vi "Convert Supported Color to .NET Color.vi"(8 "error in (no error)":errorcluster, 11 "Text Color":T1) -> (0 "error out":errorcluster, 3 ".NET Color":refnum<k24>)   [LabVIEW 2021, in "Rich Text Box.lvlib"]
uses:
  Rich Text Box.lvlib
  Text Colors.ctl
  System.Drawing
panel:
  # "see the License on the block diagram (Ctrl+E or Window:Show Block Diagram)"
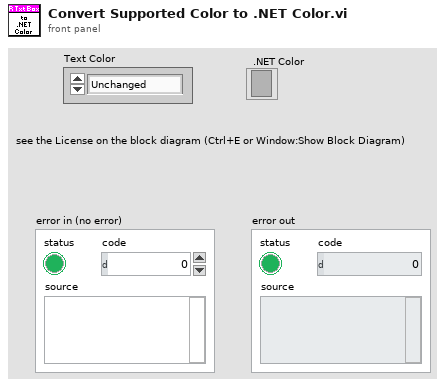
[diagram p1: front panel]
types:
  T1 = typedef "Rich Text Box.lvlib/Text Colors.ctl" = enum16{"Unchanged", "Black", "Blue", "Cyan", "Maroon", "Gray", "Violet", "Green", "Light Green", "Orange", "Yellow", "Magenta", "Red", "White"}
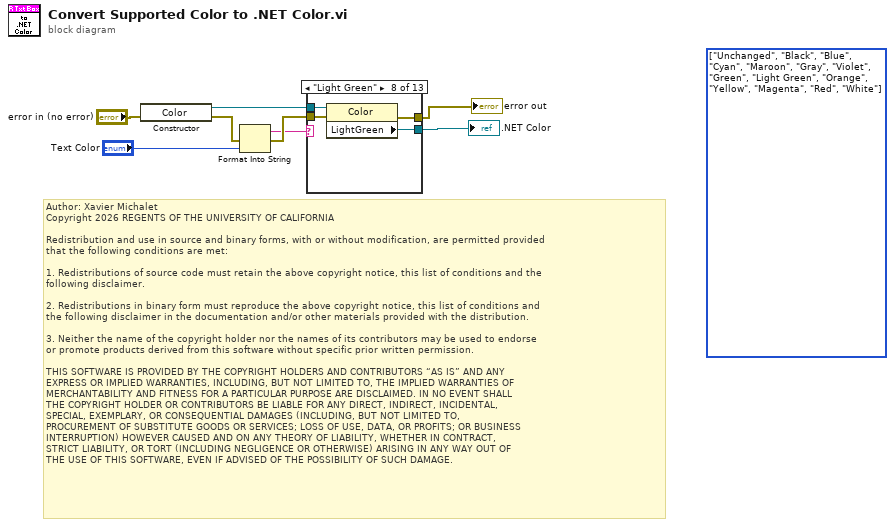
[diagram p0: block diagram]
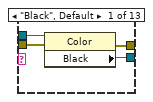
[diagram p2: hidden frame]
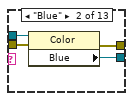
[diagram p3: hidden frame]
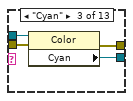
[diagram p4: hidden frame]
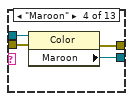
[diagram p5: hidden frame]
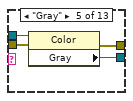
[diagram p6: hidden frame]
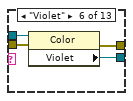
[diagram p7: hidden frame]
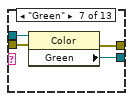
[diagram p8: hidden frame]
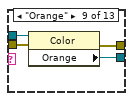
[diagram p9: hidden frame]
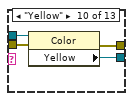
[diagram p10: hidden frame]
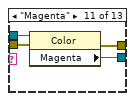
[diagram p11: hidden frame]
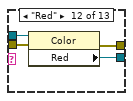
[diagram p12: hidden frame]
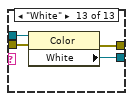
[diagram p13: hidden frame]
diagram:
  (unwired) T1[] [enum."Unchanged", enum."Black", enum."Blue", enum."Cyan", enum."Maroon", enum."Gray", enum."Violet", enum."Green", enum."Light Green", enum."Orange", enum."Yellow", enum."Magenta", enum."Red", enum."White"] items=["Unchanged", "Black", "Blue", "Cyan", "Maroon", "Gray", "Violet", "Green", "Light Green", "Orange", "Yellow", "Magenta", "Red", "White"] ("Array")
  # "Author: Xavier Michalet\nCopyright 2026 REGENTS OF THE UNIVERSITY OF CALIFORNIA\n\nRedistribution and use in source and binary forms, with or without modification, are permitted provided\nthat the following conditions are met:\n\n1. Redistributions of source code must retain the above copyright notice, this list of conditions and the\nfollowing disclaimer.\n\n2. Redistributions in binary form must reproduce the above copyright notice, this list of conditions and\nthe following disclaimer in the documentation and/or other materials provided with the distribution.\n\n3. Neither the name of the copyright holder nor the names of its contributors may be used to endorse \nor promote products derived from this software without specific prior written permission.\n\nTHIS SOFTWARE IS PROVIDED BY THE COPYRIGHT HOLDERS AND CONTRIBUTORS “AS IS” AND ANY \nEXPRESS OR IMPLIED WARRANTIES, INCLUDING, BUT NOT LIMITED TO, THE IMPLIED WARRANTIES OF\nMERCHANTABILITY AND FITNESS FOR A PARTICULAR PURPOSE ARE DISCLAIMED. IN NO EVENT SHALL\nTHE COPYRIGHT HOLDER OR CONTRIBUTORS BE LIABLE FOR ANY DIRECT, INDIRECT, INCIDENTAL, \nSPECIAL, EXEMPLARY, OR CONSEQUENTIAL DAMAGES (INCLUDING, BUT NOT LIMITED TO, \nPROCUREMENT OF SUBSTITUTE GOODS OR SERVICES; LOSS OF USE, DATA, OR PROFITS; OR BUSINESS\nINTERRUPTION) HOWEVER CAUSED AND ON ANY THEORY OF LIABILITY, WHETHER IN CONTRACT, \nSTRICT LIABILITY, OR TORT (INCLUDING NEGLIGENCE OR OTHERWISE) ARISING IN ANY WAY OUT OF\nTHE USE OF THIS SOFTWARE, EVEN IF ADVISED OF THE POSSIBILITY OF SUCH DAMAGE."
  n1 = constructor class="Color"(error in="error in (no error)") -> (reference out=w3:refnum<k24>, error out=w7:errorcluster)  [unwired: 2 in, 1 out]
  n2 = Format Into String(error in=w7, "Text Color") -> (resulting string=w5:string, error out=w8:errorcluster)  [unwired: 2 in]
  n3 = case shown="\"Light Green\"" w5 {
    tunnel: w3 -> [w12 w16 w20 w24 w28 w32 w36 w40 w44 w48 w52 w56 w60]
    tunnel: w8 -> [w11 w15 w19 w23 w27 w31 w35 w39 w43 w47 w51 w55 w59]
    tunnel: [w10 w14 w18 w22 w26 w30 w34 w38 w42 w46 w50 w54 w58] -> w2
    tunnel: [w9 w13 w17 w21 w25 w29 w33 w37 w41 w45 w49 w53 w57] -> w1
    frame "Black", Default {
      n4 = property class="Color"(reference=w12, error in=w11) -> (error out=w9:errorcluster, "Black"=w10:refnum<k24>)  [unwired: 1 out]
    }
    frame "Blue" {
      n5 = property class="Color"(reference=w16, error in=w15) -> (error out=w13:errorcluster, "Blue"=w14:refnum<k24>)  [unwired: 1 out]
    }
    frame "Cyan" {
      n6 = property class="Color"(reference=w20, error in=w19) -> (error out=w17:errorcluster, "Cyan"=w18:refnum<k24>)  [unwired: 1 out]
    }
    frame "Maroon" {
      n7 = property class="Color"(reference=w24, error in=w23) -> (error out=w21:errorcluster, "Maroon"=w22:refnum<k24>)  [unwired: 1 out]
    }
    frame "Gray" {
      n8 = property class="Color"(reference=w28, error in=w27) -> (error out=w25:errorcluster, "Gray"=w26:refnum<k24>)  [unwired: 1 out]
    }
    frame "Violet" {
      n9 = property class="Color"(reference=w32, error in=w31) -> (error out=w29:errorcluster, "Violet"=w30:refnum<k24>)  [unwired: 1 out]
    }
    frame "Green" {
      n10 = property class="Color"(reference=w36, error in=w35) -> (error out=w33:errorcluster, "Green"=w34:refnum<k24>)  [unwired: 1 out]
    }
    frame "Light Green" {
      n11 = property class="Color"(reference=w40, error in=w39) -> (error out=w37:errorcluster, "LightGreen"=w38:refnum<k24>)  [unwired: 1 out]
    }
    frame "Orange" {
      n12 = property class="Color"(reference=w44, error in=w43) -> (error out=w41:errorcluster, "Orange"=w42:refnum<k24>)  [unwired: 1 out]
    }
    frame "Yellow" {
      n13 = property class="Color"(reference=w48, error in=w47) -> (error out=w45:errorcluster, "Yellow"=w46:refnum<k24>)  [unwired: 1 out]
    }
    frame "Magenta" {
      n14 = property class="Color"(reference=w52, error in=w51) -> (error out=w49:errorcluster, "Magenta"=w50:refnum<k24>)  [unwired: 1 out]
    }
    frame "Red" {
      n15 = property class="Color"(reference=w56, error in=w55) -> (error out=w53:errorcluster, "Red"=w54:refnum<k24>)  [unwired: 1 out]
    }
    frame "White" {
      n16 = property class="Color"(reference=w60, error in=w59) -> (error out=w57:errorcluster, "White"=w58:refnum<k24>)  [unwired: 1 out]
    }
  }
  ".NET Color" <- w2
  "error out" <- w1
